vi "Robot Drive - Begin.vi"(8 "error in (no error)":errorcluster) -> (0 "error out":errorcluster)   [LabVIEW 2015]
uses:
  <vilib>/Rock Robotics/SystemInterfaces/DIO/FPGA_DIOPWMChannel.ctl
  <vilib>/Rock Robotics/WPI/SafetyOutput/WPI_SafetyOutputConfigMenu.ctl
  <vilib>/Rock Robotics/SystemInterfaces/AI/FPGA_AIGyroChannel.ctl
  <vilib>/Rock Robotics/SystemInterfaces/AI/FPGA_AIChannel.ctl
  <vilib>/Rock Robotics/WPI/RobotDrive/WPI_RobotDriveOpen4MotorWithSPARK.vi
  <vilib>/Rock Robotics/WPI/Gyro/WPI_GyroAnalogOpen.vi
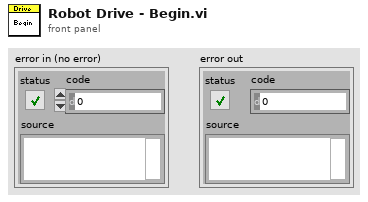
[diagram p1: front panel]
types:
  T1 = typedef "FPGA_AIChannel.ctl" = enum8{"AI 0", "AI 1", "AI 2", "AI 3", "AI MXP 0", "AI MXP 1", "AI MXP 2", "AI MXP 3", "Invalid"}
  T2 = typedef "FPGA_AIGyroChannel.ctl" = enum8{"AI 0", "AI 1", "Invalid"}
  T3 = typedef "FPGA_DIOPWMChannel.ctl" = enum8{"PWM 0", "PWM 1", "PWM 2", "PWM 3", "PWM 4", "PWM 5", "PWM 6", "PWM 7", "PWM 8", "PWM 9", "PWM MXP 0", "PWM MXP 1", "PWM MXP 2", "PWM MXP 3", "PWM MXP 4", "PWM MXP 5", "PWM MXP 6", "PWM MXP 7", "PWM MXP 8", "PWM MXP 9", "Invalid"}
  T4 = typedef "WPI_SafetyOutputConfigMenu.ctl" = enum16{"Enable", "Disable"}
  T5 = typedef "WPI_RobotDriveDevRef.ctl" = cluster{"DevStatus":errorcluster, "Motors[]":T6[], "Square Inputs":bool, "Max Output":dbl}
  T6 = typedef "WPI_MotorControlDeviceRef.ctl" = cluster{"DeviceStatus":errorcluster, "Type":T7, "PWM":cluster{"PWM Channel":T3, "DeadBand":T8}, "CAN":cluster{"Device Number":u8, "Control Mode":T9, "Semaphore":T10, "Max Vout":dbl, "TalonSRX Control Mode":T11}, "Invert":bool}
  T7 = typedef "WPI_MotorControlType.ctl" = enum16{"PWM", "CAN", "CANTalonSRX"}
  T8 = typedef "WPI_PWMDeadband.ctl" = cluster{"Name":string, "maxPositivePwm":i32, "minPositivePwm":i32, "centerPwm":i32, "maxNegativePwm":i32, "minNegativePwm":i32, "angularRange":u16}
  T9 = typedef "WPI_CANJaguar_ControlMode.ctl" = enum8{"Percent VBus", "Current", "Speed", "Position", "Voltage"}
  T10 = typedef "Semaphore RefNum" = refnum<k1>
  T11 = typedef "WPI_CANTalonSRX_APIControlMode.ctl" = enum8{"Percent VBus", "Speed", "Position", "Slave", "Unchanged / Invalid", "Voltage Compensation", "Current", "Motion Profile"}
  T12 = typedef "WPI_GyroDevRef.ctl" = cluster{"DevStatus":errorcluster, "Analog Channel":T1, "Offset":dbl, "Gain (VoltsPerDegree/Second)":dbl, "Gyro Type":enum16{"Analog", "XRS450"}, "Handle":i32, "SPI Bus":T13, "Device Found":bool, "Sample Rate":dbl, "Calibrate On Open":bool}
  T13 = typedef "spi_bus.ctl" = enum16{"SPI On-Board, CS0", "SPI On-Board, CS1", "SPI On-Board, CS2", "SPI On-Board, CS3", "SPI MXP", "Invalid"}
  T14 = typedef "WPI_AnalogChannelDevRef.ctl" = cluster{"DevStatus":errorcluster, "Analog Channel":T1}
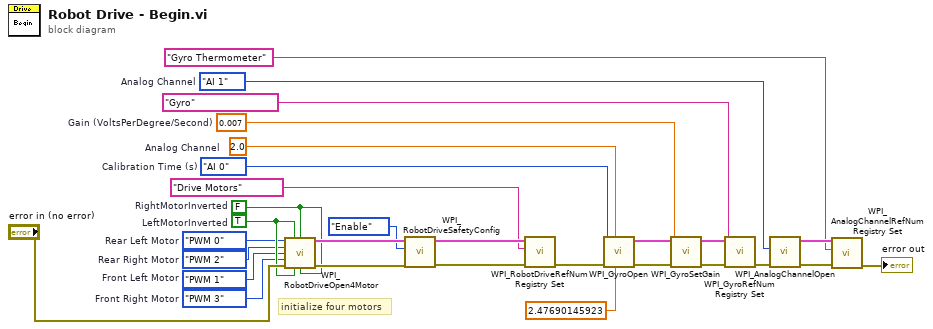
[diagram p0: block diagram]
diagram:
  w6 = FPGA_AIChannel."AI 1"  # Analog Channel
  w8 = 0.007  # Gain (VoltsPerDegree/Second)
  w14 = 2.0  # Calibration Time (s)
  w15 = FPGA_AIGyroChannel."AI 0"  # Analog Channel
  w22 = FPGA_DIOPWMChannel."PWM 3"  # Front Right Motor
  w21 = FPGA_DIOPWMChannel."PWM 1"  # Front Left Motor
  w19 = FPGA_DIOPWMChannel."PWM 2"  # Rear Right Motor
  w18 = FPGA_DIOPWMChannel."PWM 0"  # Rear Left Motor
  w23 = TRUE  # LeftMotorInverted
  w24 = FALSE  # RightMotorInverted
  # "initialize four motors"
  n1 = call-poly <vilib>:"WPI_RobotDriveOpen4Motor.vi"("Rear Left Motor"=w18, "Rear Left Motor Inverted"=w23, "Rear Right Motor Inverted"=w24, "Rear Right Motor"=w19, "Front Left Motor"=w21, "Front Right Motor"=w22, "error in (no error)"="error in (no error)", "Front Left Motor Inverted"=w23, "Front Right Motor Inverted"=w24) -> ("RobotDriveDevRef"=w26:T5, "error out"=w27:errorcluster)  [unwired: 5 in]
  n2 = call <vilib>:"WPI_RobotDriveSafetyConfig.vi"("error in (no error)"=w27, "mode"=WPI_SafetyOutputConfigMenu."Enable", "RobotDriveDevRef"=w26) -> ("error out"=w28:errorcluster, "RobotDriveDevRef"=w29:T5)  [unwired: 7 in]
  n3 = call <vilib>:"WPI_RobotDriveRefNum Registry Set.vi"("error in (no error)"=w28, "refnum name"="Drive Motors", "RobotDriveDevRef"=w29) -> ("error out"=w16:errorcluster)  [unwired: 1 in, 7 out]
  n4 = call-poly <vilib>:"WPI_GyroOpen.vi"("Calibrated Center Voltage"=2.47690145923, "Calibration Time (s)"=w14, "error in (no error)"=w16, "Analog Channel"=w15) -> ("error out"=w11:errorcluster, "GyroDevRef"=w12:T12)  [unwired: 5 in, 1 out]
  n5 = call <vilib>:"WPI_GyroSetGain.vi"("error in (no error)"=w11, "Gain (VoltsPerDegree/Second)"=w8, "GyroDevRef"=w12) -> ("error out"=w9:errorcluster, "GyroDevRef"=w10:T12)  [unwired: 7 in]
  n6 = call <vilib>:"WPI_GyroRefNum Registry Set.vi"("error in (no error)"=w9, "refnum name"="Gyro", "GyroDevRef"=w10) -> ("error out"=w7:errorcluster)  [unwired: 7 in, 1 out]
  n7 = call <vilib>:"WPI_AnalogChannelOpen.vi"("error in (no error)"=w7, "Analog Channel"=w6) -> ("error out"=w5:errorcluster, "AIDeviceRef"=w4:T14)  [unwired: 8 in]
  n8 = call <vilib>:"WPI_AnalogChannelRefNum Registry Set.vi"("error in (no error)"=w5, "refnum name"="Gyro Thermometer", "AIDeviceRef"=w4) -> ("error out"=→"error out":errorcluster)  [unwired: 7 in, 1 out]
